vi "GetInitialTemperature.vi"(9 "level":dbl, 10 "room_temperature":dbl, 11 "tank_resolution":T1) -> (3 "initial_temperature":dbl[][](array[numeric]))   [LabVIEW 2020]
uses:
  TankResolution.ctl
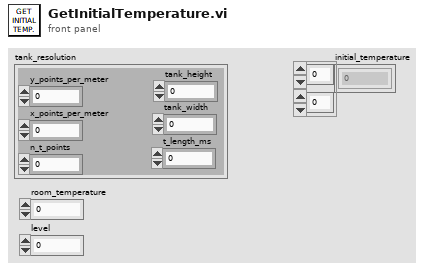
[diagram p1: front panel]
types:
  T1 = typedef "TankResolution.ctl" = cluster{"y_points_per_meter":i32, "x_points_per_meter":i32, "n_t_points":i32, "tank_height":dbl, "tank_width":dbl, "t_length_ms":u32}
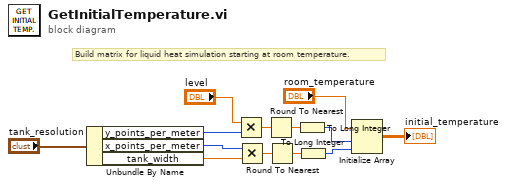
[diagram p0: block diagram]
diagram:
  # "Build matrix for liquid heat simulation starting at room temperature."
  n1 = Unbundle By Name("tank_resolution") -> ("y_points_per_meter"=w4:i32, "x_points_per_meter"=w9:i32, "tank_width"=w10:dbl)
  n2 = Multiply(x="level", y=w4) -> (x*y=w2:dbl)
  n3 = Multiply(x=w9, y=w10) -> (x*y=w7:dbl)
  n4 = Round To Nearest(number=w2) -> (nearest integer value=w3:dbl)
  n5 = Round To Nearest(number=w7) -> (nearest integer value=w6:dbl)
  n6 = To Long Integer(number=w3) -> (32bit integer=w5:i32)
  n7 = To Long Integer(number=w6) -> (32bit integer=w8:i32)
  n8 = Initialize Array("room_temperature", w5, w8) -> (→"initial_temperature":dbl[][])
